vi "Animacion(conSprites).vi"() -> ()   [LabVIEW 2017]
uses:
  <vilib>/picture/picture.llb/Draw True-Color Pixmap.vi
panel:
  in  "i(sprite)":i16=8
  in  "Donde?":cluster{"x":i16, "y":i16}
  out "Mundo2":picture
  # "y=214"
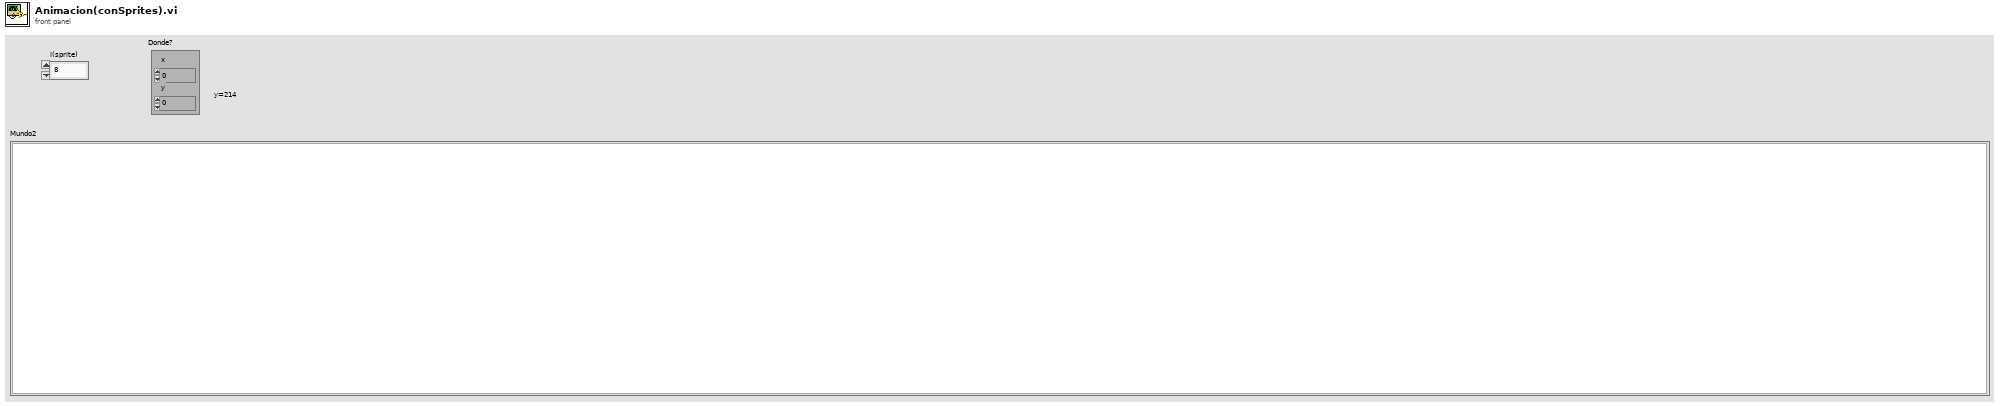
[diagram p1: front panel]
types:
  T1 = typedef "imagedata.ctl" = cluster{"image type":i32, "image depth":i32, "image":u8[], "mask":u8[], "colors":u32[], "Rectangle":cluster{"left":i16, "top":i16, "right":i16, "bottom":i16}}
  T2 = cluster{"left":i16, "top":i16, "right":i16, "bottom":i16}
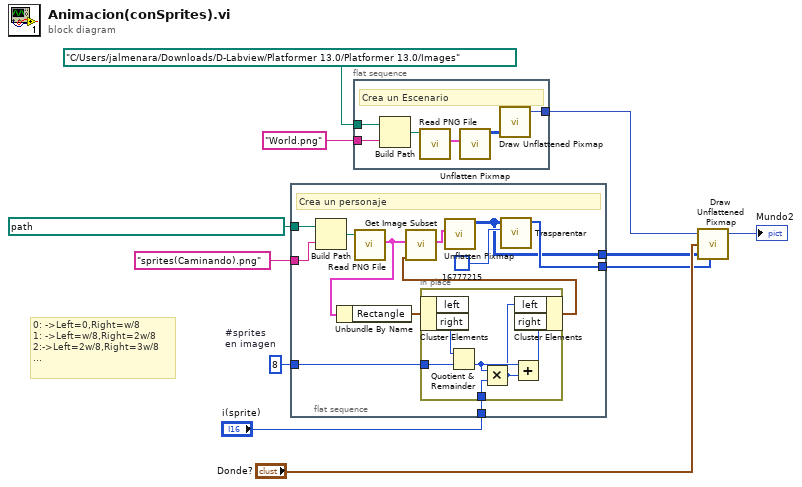
[diagram p0: block diagram]
diagram:
  w7 = i16 8  # #sprites en imagen
  # "0: ->Left=0,Right=w/8\n1: ->Left=w/8,Right=2w/8\n2:->Left=2w/8,Right=3w/8\n..."
  n1 = flat-sequence {
    tunnel: path "F:/Prog/LabVIEW/Pruebas/Animación/con sprites" ("path to PNG file") -> [w23]
    tunnel: "sprites(Caminando).png" ("format string") -> [w22]
    tunnel: w7 -> [w17]
    tunnel: "i(sprite)" -> [w16]
    tunnel: [w14] -> w3
    tunnel: [w13] -> w2
    frame #0 {
      # "Crea un personaje"
      n2 = Build Path(base path=w23, name or relative path=w22) -> (appended path=w21:path)
      n3 = call <vilib>:"Read PNG File.vi"("path to PNG file"=w21) -> ("image data"=w20:T1)  [unwired: 8 in, 2 out]
      n4 = Unbundle By Name(w20) -> ("Rectangle"=w18:T2)
      n5 = in-place {
        in-place-border: w17 -> [w29]
        in-place-border: w16 -> [w27]
        n6 = in-place-cluster #1(w18) -> ("right"=w28:i16)  [unwired: 1 out]
        n7 = Quotient & Remainder(x=w28, y=w29) -> (floor(x/y)=w26:i16)  [unwired: 1 out]
        n8 = Multiply(x=w26, y=w27) -> (x*y=w24:i16)
        n9 = Add(x=w26, y=w24) -> (x+y=w25:i16)
        n10 = in-place-cluster #1("left"=w24, "right"=w25) -> (w19:T2)
      }
      n11 = call <vilib>:"Get Image Subset.vi"("subset rect"=w19, "image data"=w20) -> ("image subset"=w12:T1)  [unwired: 4 in, 1 out]
      n12 = call <vilib>:"Unflatten Pixmap.vi"("image data"=w12) -> ("24-bit pixmap"=w13:u32[][])  [unwired: 4 in, 6 out]
      n13 = call "Trasparentar.vi"("Background Color"=u32 16777215, "24-bit pixmap"=w13) -> ("Mask"=w14:u8[])  [unwired: 9 in]
    }
  }
  n14 = flat-sequence {
    tunnel: "World.png" ("format string") -> [w34]
    tunnel: path "C:/Users/jalmenara/Downloads/D-Labview/Platformer 13.0/Platformer 13.0/Images" ("path to PNG file") -> [w33]
    tunnel: [w31] -> w1
    frame #0 {
      # "Crea un Escenario"
      n15 = Build Path(base path=w33, name or relative path=w34) -> (appended path=w32:path)
      n16 = call <vilib>:"Read PNG File.vi"("path to PNG file"=w32) -> ("image data"=w35:T1)  [unwired: 8 in, 2 out]
      n17 = call <vilib>:"Unflatten Pixmap.vi"("image data"=w35) -> ("24-bit pixmap"=w30:u32[][])  [unwired: 4 in, 6 out]
      n18 = call-poly <vilib>:"Draw Unflattened Pixmap.vi"("data (RGB format)"=w30) -> ("new picture"=w31:picture)  [unwired: 8 in]
    }
  }
  n19 = call-poly <vilib>:"Draw Unflattened Pixmap.vi"("picture"=w1, "top left point(0, 0)"="Donde?", "data (RGB format)"=w2, "mask"=w3) -> ("new picture"=→"Mundo2":picture)  [unwired: 5 in]
